vi "Ex2_NumericCaseStructure.vi"() -> ()   [LabVIEW 2024]
panel:
  in  "OK Button":dbl
  in  "OK Button 2":bool
  out "Numeric 3":dbl
  in  "Numeric 2":dbl
  in  "Numeric":dbl
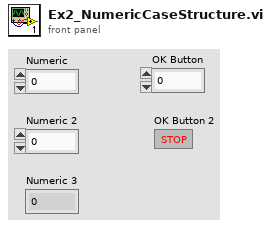
[diagram p1: front panel]
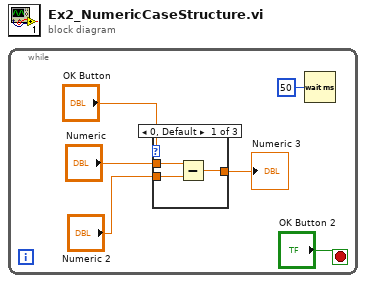
[diagram p0: block diagram]
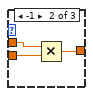
[diagram p2: hidden frame]
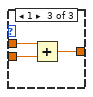
[diagram p3: hidden frame]
diagram:
  n1 = while {
    stop <- "OK Button 2" stop-if-true
    n2 = case shown="0, Default" "OK Button" {
      tunnel: "Numeric 2" -> [w7 w10 w15]
      tunnel: "Numeric" -> [w8 w11 w14]
      tunnel: [w9 w12 w13] -> w4
      frame 0, Default {
        n3 = Subtract(x=w8, y=w7) -> (x-y=w9:dbl)
      }
      frame -1 {
        n4 = Multiply(x=w11, y=w10) -> (x*y=w12:dbl)
      }
      frame 1 {
        n5 = Add(x=w14, y=w15) -> (x+y=w13:dbl)
      }
    }
    "Numeric 3" <- w4
    n6 = Wait (ms)(milliseconds to wait=u32 50) -> ()  [unwired: 1 out]
  }
